vi "Write channel pattern matches.vi"(8 "error in (no error)":errorcluster, 10 "channel pattern matches":string[](array[string]), 11 "TDMS datalogger configuration in":refnum<class "TDMS datalogger configuration.lvclass">) -> (0 "error out":errorcluster, 3 "TDMS datalogger configuration out":refnum<class "TDMS datalogger configuration.lvclass">)   [LabVIEW 2013, in "TDMS datalogger configuration.lvclass"]
uses:
  TDMS datalogger configuration.lvclass
  TDMS datalogger configuration.lvclass/TDMS datalogger configuration.ctl
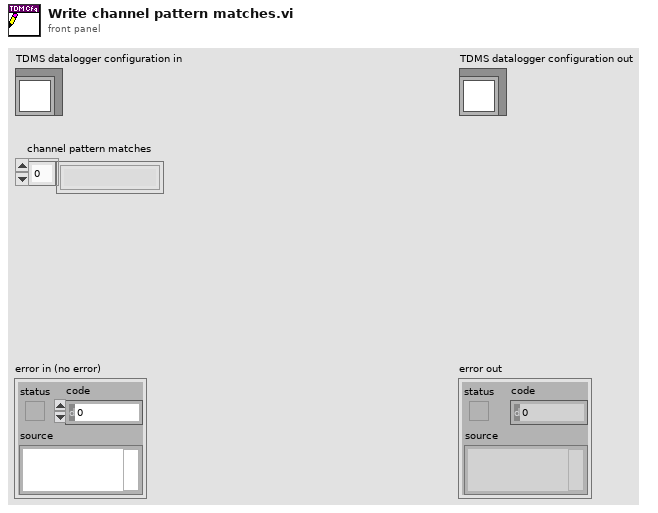
[diagram p1: front panel]
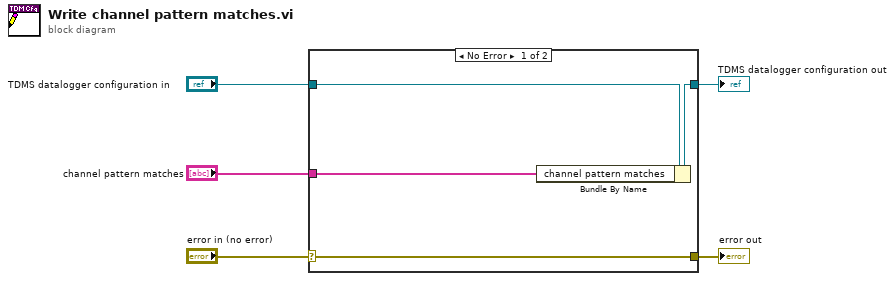
[diagram p0: block diagram]
diagram:
  n1 = case shown="No Error" "error in (no error)" {
    selector: "error in (no error)" -> [w9 w10]
    tunnel: [w9 w10] -> w4
    tunnel: [w7 w11] -> w2
    tunnel: "TDMS datalogger configuration in" -> [w8 w11]
    tunnel: "channel pattern matches" -> [w6 _]
    frame No Error {
      n2 = Bundle By Name(cluster=w8, "channel pattern matches"=w6) -> (w7:refnum<class "TDMS datalogger configuration.lvclass">)
    }
    frame Error {
    }
  }
  "error out" <- w4
  "TDMS datalogger configuration out" <- w2
